vi "AddSequenceStartCondition.vi"(8 "error in (no error)":errorcluster, 9 "Number of Samples In":i32, 10 "Data Array In":u8[][](array[numeric]), 11 "RFFE_Data In":T1 {"Toggle (high to low)" items=["0", "1", "Z", "L", "H", "X", "T", "V"]; "X Array" items=["0", "1", "Z", "L", "H", "X", "T", "V"]; "Z Array" items=["0", "1", "Z", "L", "H", "X", "T", "V"]; "L Array" items=["0", "1", "Z", "L", "H", "X", "T", "V"]; "H Array" items=["0", "1", "Z", "L", "H", "X", "T", "V"]; "One Array" items=["0", "1", "Z", "L", "H", "X", "T", "V"]; "Zero Array" items=["0", "1", "Z", "L", "H", "X", "T", "V"]}) -> (0 "error out":errorcluster, 1 "Number of Samples Out":i32, 2 "Data Array Out":u8[][](array[numeric]), 3 "RFFE_Data Out":T1 {"Toggle (high to low)" items=["0", "1", "Z", "L", "H", "X", "T", "V"]; "X Array" items=["0", "1", "Z", "L", "H", "X", "T", "V"]; "Z Array" items=["0", "1", "Z", "L", "H", "X", "T", "V"]; "L Array" items=["0", "1", "Z", "L", "H", "X", "T", "V"]; "H Array" items=["0", "1", "Z", "L", "H", "X", "T", "V"]; "One Array" items=["0", "1", "Z", "L", "H", "X", "T", "V"]; "Zero Array" items=["0", "1", "Z", "L", "H", "X", "T", "V"]})   [LabVIEW 2013]
doc: "Builds a MIPI RFFE sequence start condition."
uses:
  Ctrls/RFFE_Data.ctl
  Ctrls/ClockDataChannels.ctl
  Ctrls/BitStates.ctl
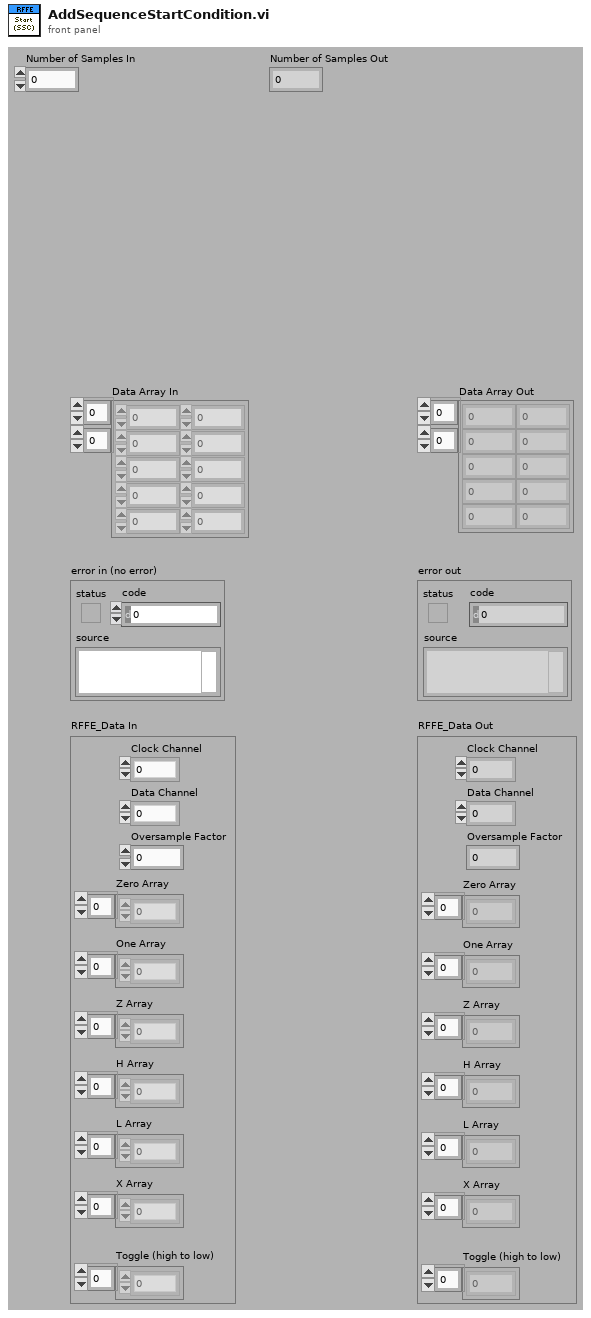
[diagram p1: front panel]
types:
  T1 = typedef "RFFE_Data.ctl" = cluster{"Clock Channel":T2, "Data Channel":T2, "Oversample Factor":u8, "Zero Array":u8[], "One Array":u8[], "Z Array ":u8[], "H Array":u8[], "L Array":u8[], "X Array":u8[], "Toggle (high to low)":u8[]}
  T2 = typedef "ClockDataChannels.ctl" = enum16{"0", "1"}
  T3 = typedef "BitStates.ctl" = enum16{"0", "1", "Z", "L", "H", "X", "Toggle"}
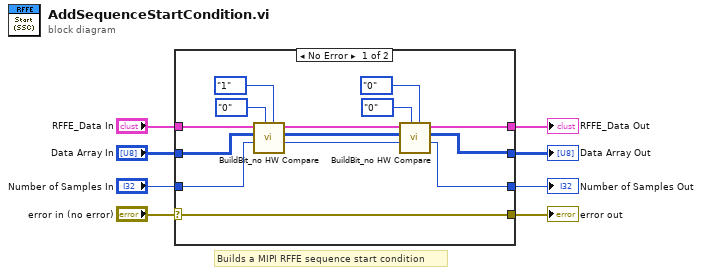
[diagram p0: block diagram]
diagram:
  # "Builds a MIPI RFFE sequence start condition"
  n1 = case shown="No Error" "error in (no error)" {
    selector: "error in (no error)" -> [w22 w26]
    tunnel: [w22 w26] -> w7
    tunnel: [w10 w25] -> w6
    tunnel: "RFFE_Data In" -> [w15 w25]
    tunnel: [w11 w24] -> w5
    tunnel: "Data Array In" -> [w21 w24]
    tunnel: "Number of Samples In" -> [w20 w23]
    tunnel: [w12 w23] -> w1
    frame No Error {
      n2 = call "BuildBit_no HW Compare.vi"("Data Value"=BitStates."1", "Clock Value"=BitStates."0", "Number of Samples In"=w20, "Data Array In"=w21, "RFFE_Data In"=w15) -> ("Number of Samples Out"=w13:i32, "Data Array Out"=w14:u8[][], "RFFE_Data Out"=w9:T1)  [unwired: 4 in]
      n3 = call "BuildBit_no HW Compare.vi"("Data Value"=BitStates."0", "Clock Value"=BitStates."0", "Number of Samples In"=w13, "Data Array In"=w14, "RFFE_Data In"=w9) -> ("Number of Samples Out"=w12:i32, "Data Array Out"=w11:u8[][], "RFFE_Data Out"=w10:T1)  [unwired: 4 in]
    }
    frame Error {
    }
  }
  "error out" <- w7
  "RFFE_Data Out" <- w6
  "Data Array Out" <- w5
  "Number of Samples Out" <- w1
